vi "State.vi"(11 "Entity in":refnum<class "Entity.lvclass">) -> (2 "Entity State":T1)   [LabVIEW 2020, in "Conditum.lvlib" / "Entity.lvclass"]
uses:
  Entity.lvclass
  Entity.lvclass/Entity.ctl
  Entity State.ctl
  Conditum.lvlib
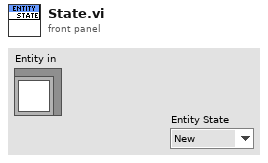
[diagram p1: front panel]
types:
  T1 = typedef "Conditum.lvlib/Entity State.ctl" = enum16{"New", "Managed", "Detached", "Removed"}
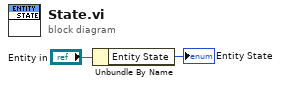
[diagram p0: block diagram]
diagram:
  n1 = Unbundle By Name("Entity in") -> ("Entity State"=→"Entity State":T1)
